vi "Receive U8x2 CMD and String Data.vi"(0 "TCP Ref In":refnum<k5>, 1 "Time Out(ms)":i32=100, 11 "error in (no error)":errorcluster) -> (4 "TCP Ref Out":refnum<k5>, 6 "High CMD":u8, 8 "Low CMD":u8, 10 "Data":string, 15 "error out":errorcluster)   [LabVIEW 2024]
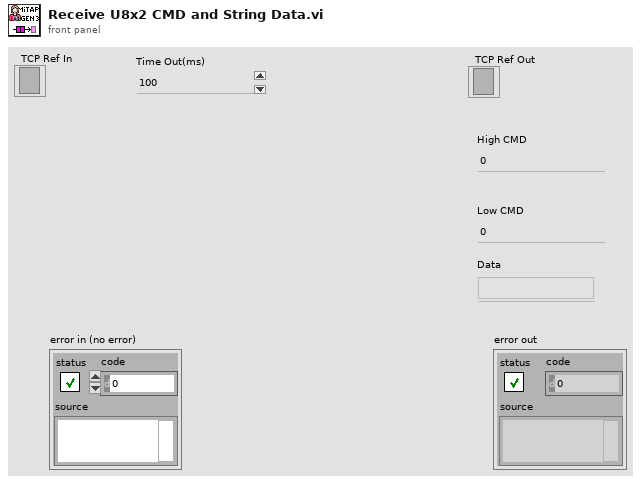
[diagram p1: front panel]
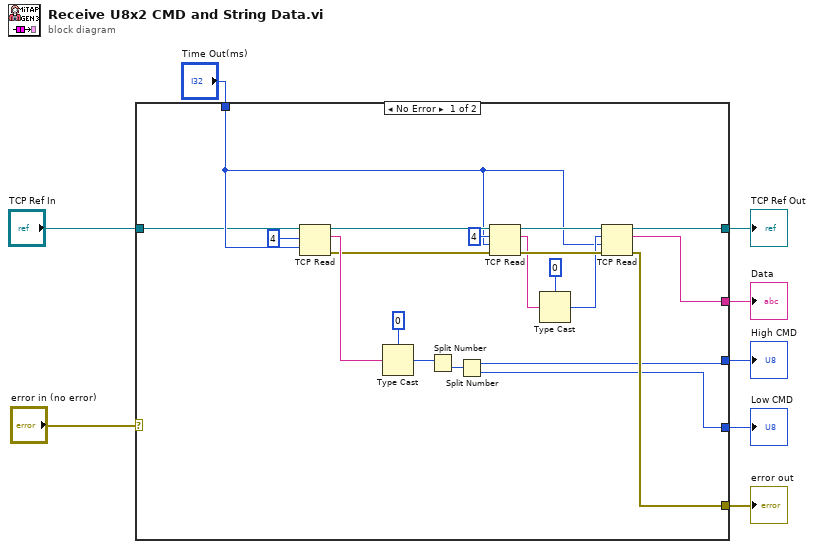
[diagram p0: block diagram]
diagram:
  n1 = case shown="No Error" "error in (no error)" {
    selector: "error in (no error)" -> [_ w30]
    tunnel: [w12 w30] -> w7
    tunnel: [w9 _] -> w6
    tunnel: [w17 _] -> w5
    tunnel: "Time Out(ms)" -> [w16 _]
    tunnel: "TCP Ref In" -> [w15 w29]
    tunnel: [w14 w29] -> w2
    tunnel: [w11 _] -> w1
    frame No Error {
      n2 = TCP Read(connection ID=w15, bytes to read=4, 9:w16) -> (connection ID out=w27:refnum<k5>, data out=w26:string, error out=w24:errorcluster)  [unwired: 2 in]
      n3 = Type Cast(type=u32 0 ("bytes to read"), x=w26) -> (*(type *) &x=w10:u32)
      n4 = Split Number(x=w10) -> (lo(x)=w13:u16)  [unwired: 1 out]
      n5 = Split Number(x=w13) -> (hi(x)=w9:u8, lo(x)=w11:u8)
      n6 = TCP Read(connection ID=w27, bytes to read=4, error in (no error)=w24, 9:w16) -> (connection ID out=w21:refnum<k5>, data out=w19:string, error out=w22:errorcluster)  [unwired: 1 in]
      n7 = Type Cast(type=0 ("bytes to read"), x=w19) -> (*(type *) &x=w18:i32)
      n8 = TCP Read(connection ID=w21, bytes to read=w18, error in (no error)=w22, 9:w16) -> (connection ID out=w14:refnum<k5>, data out=w17:string, error out=w12:errorcluster)  [unwired: 1 in]
    }
    frame Error {
    }
  }
  "error out" <- w7
  "High CMD" <- w6
  "Data" <- w5
  "TCP Ref Out" <- w2
  "Low CMD" <- w1
